vi "Bundle.vi"(7 "Await Completion?(F)":bool, 8 "error in (no error)":errorcluster, 9 "Perform Post Actions?(T)":bool=TRUE, 10 "File Post Action":refnum<class "File Post Action.lvclass">[](array[class]), 11 "Close File Msg in":refnum<class "Close File Msg.lvclass">) -> (0 "error out":errorcluster, 3 "Close File Msg out":refnum<class "Close File Msg.lvclass">)   [LabVIEW 2020, in "File Writer.lvlib" / "Close File Msg.lvclass"]
doc: "Write File Post Actions and the Perform Post Actions to the private data."
uses:
  Close File Msg.lvclass
  File Writer/File Post Action/File Post Action.lvclass
  Close File Msg.lvclass/Close File Msg.ctl
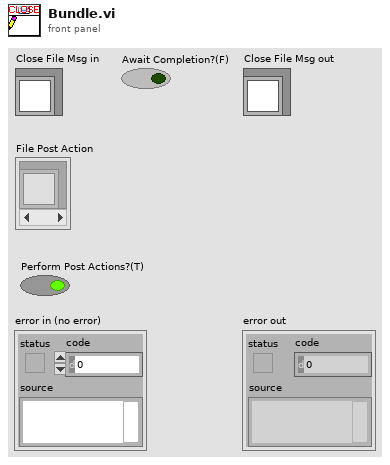
[diagram p1: front panel]
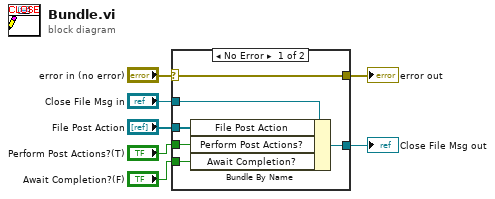
[diagram p0: block diagram]
diagram:
  n1 = case shown="No Error" "error in (no error)" {
    selector: "error in (no error)" -> [w13 w14]
    tunnel: [w13 w14] -> w6
    tunnel: [w11 w15] -> w4
    tunnel: "Close File Msg in" -> [w12 w15]
    tunnel: "File Post Action" -> [w10 _]
    tunnel: "Perform Post Actions?(T)" -> [w9 _]
    tunnel: "Await Completion?(F)" -> [w8 _]
    frame No Error {
      n2 = Bundle By Name(cluster=w12, "File Post Action"=w10, "Perform Post Actions?"=w9, "Await Completion?"=w8) -> (w11:refnum<class "Close File Msg.lvclass">)
    }
    frame Error {
    }
  }
  "error out" <- w6
  "Close File Msg out" <- w4
